vi "_RT_CtrlLoop_Interrupt_Program.vi"(8 "error in (no error)":errorcluster) -> (0 "error out":errorcluster)   [LabVIEW 2018]
uses:
  PublicSubVI/Ctl/_ctl_RT_Working_State.ctl
  PublicSubVI/Ctl/_ctl_RT_SysLog.ctl
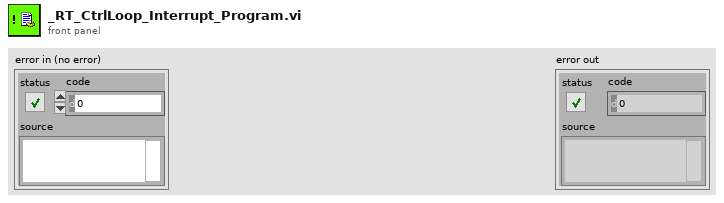
[diagram p1: front panel]
types:
  T1 = typedef "_ctl_RT_SysLog.ctl" = enum16{"None", "Initialize", "StartupRT", "StartupFPGA", "StartupAllocator", "GetMass", "SetWfmCode", "SetLaserCtrl", "SetTurboCtrl", "SetD999Ctrl", "Reconnecting...", "Interrupt", "StopRT"}
  T2 = typedef "_ctl_RT_Working_State.ctl" = enum16{"Initialize", "Running", "Reboot_Work", "Reboot_Safe"}
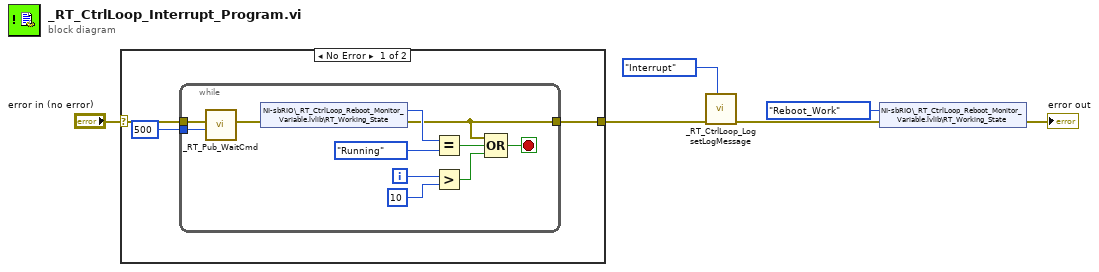
[diagram p0: block diagram]
diagram:
  n1 = case shown="No Error" "error in (no error)" {
    selector: "error in (no error)" -> [w7 w21]
    tunnel: [w8 w21] -> w5
    frame No Error {
      n2 = while {
        tunnel: u32 500 ("milliseconds to wait") -> [w16]
        tunnel: [w14] -> w8
        tunnel: w7 -> [w10]
        i -> [w18]
        stop <- w11 stop-if-true
        n3 = call "_RT_Pub_WaitCmd.vi"("milliseconds to wait"=w16, "error in (no error)"=w10) -> ("error out"=w15:errorcluster)  [unwired: 9 in]
        n4 = shared-variable "NI-sbRIO\\_RT_CtrlLoop_Reboot_Monitor_Variable.lvlib\\RT_Working_State"(error in=w15) -> (w20:T2, error out=w14:errorcluster)
        n5 = Equal?(x=w20, y=_ctl_RT_Working_State."Running") -> (x = y?=w13:bool)
        n6 = Greater?(x=w18, y=10) -> (0:w12:bool)
        n7 = Compound Arithmetic op=OR(w14, w13, w12) -> (w11:bool)
      }
    }
    frame Error {
    }
  }
  n8 = call "_RT_CtrlLoop_Log setLogMessage.vi"("system type"=_ctl_RT_SysLog."Interrupt", "error in"=w5) -> ("error out"=w4:errorcluster)  [unwired: 8 in, 1 out]
  n9 = shared-variable "NI-sbRIO\\_RT_CtrlLoop_Reboot_Monitor_Variable.lvlib\\RT_Working_State"(_ctl_RT_Working_State."Reboot_Work" ("RT_Working_State"), error in=w4) -> (error out=→"error out":errorcluster)
